vi "Get Data_old.vi"(8 "error in":errorcluster, 11 "PPT in":refnum<class "PPT.lvclass">) -> (0 "error out":errorcluster, 2 "DataOut":refnum<class "Single_Array.lvclass">, 3 "PPT out":refnum<class "PPT.lvclass">)   [LabVIEW 2014, in "PPT.lvclass"]
uses:
  PPT.lvclass
  Reusable/Data/Array Data/Single 1-D/Single_Array.lvclass
  Reusable/Data/Array Data/Single 1-D/Write Data.vi
  Reusable/Data/Write measTime.vi
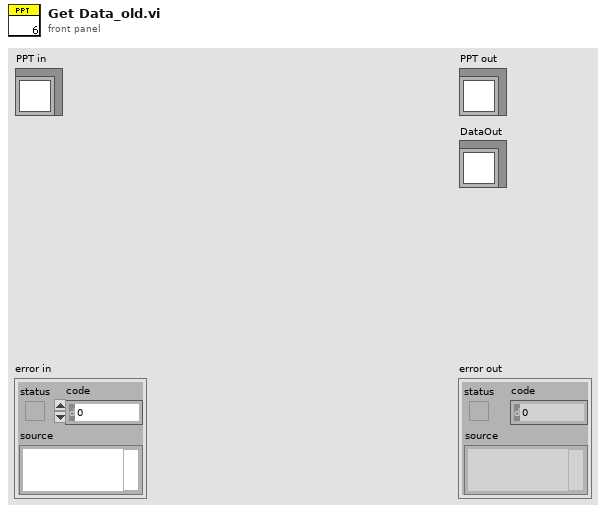
[diagram p1: front panel]
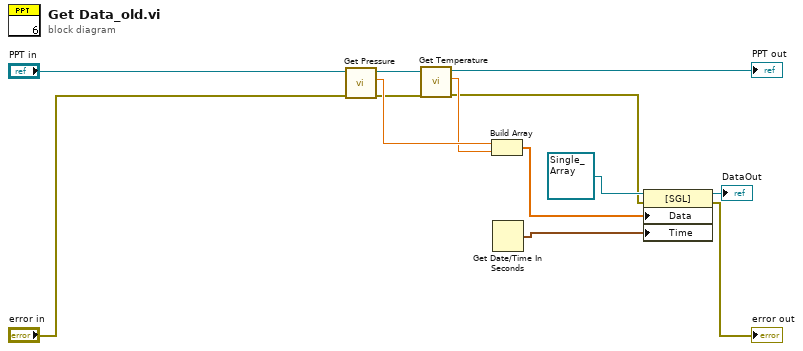
[diagram p0: block diagram]
diagram:
  n1 = call "Get Pressure.vi"("error in (no error)"="error in", "PPT in"="PPT in") -> ("error out"=w3:errorcluster, "P"=w9:dbl, "PPT out"=w13:refnum<class "PPT.lvclass">)  [unwired: 7 in]
  n2 = call "Get Temperature.vi"("error in (no error)"=w3, "PPT in"=w13) -> ("error out"=w2:errorcluster, "T"=w8:dbl, "PPT out"=→"PPT out":refnum<class "PPT.lvclass">)  [unwired: 7 in]
  n3 = Build Array(w9, w8) -> (w7:dbl[])
  n4 = Get Date/Time In Seconds() -> (seconds since 1Jan1904=w6:timestamp)
  n5 = property class="[SGL]"(reference=refnum<class "Single_Array.lvclass"> refnum ("Base Data Lib:[SGL]"), error in=w2, "Data"=w7, "Time"=w6) -> (reference out=→"DataOut":refnum<class "Single_Array.lvclass">, error out=→"error out":errorcluster)
